vi "Parse Diff Report to Text.vi"(0 "XML Path":path, 1 "Ignore cosmetic changes? (T)":bool=TRUE, 11 "error in":errorcluster) -> (4 "change description":string, 15 "error out":errorcluster)   [LabVIEW 2020, in "Graphical Diff.lvlib"]
uses:
  Graphical Diff.lvlib
  <vilib>/xml/NI_XML.lvlib
  <resource>/objmgr/DOMUserDefRef.rc
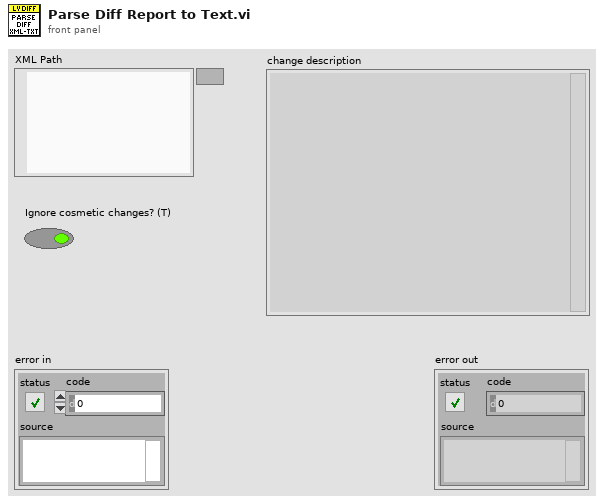
[diagram p1: front panel]
types:
  T1 = cluster{"Value":string, "Value":string, "Value":string, "Value":string}
  T2 = cluster{"Value":string, "Value":string, "Value":string, "Value":string}[]
  T3 = cluster{string, cluster{"Value":string, "Value":string, "Value":string, "Value":string}[]}
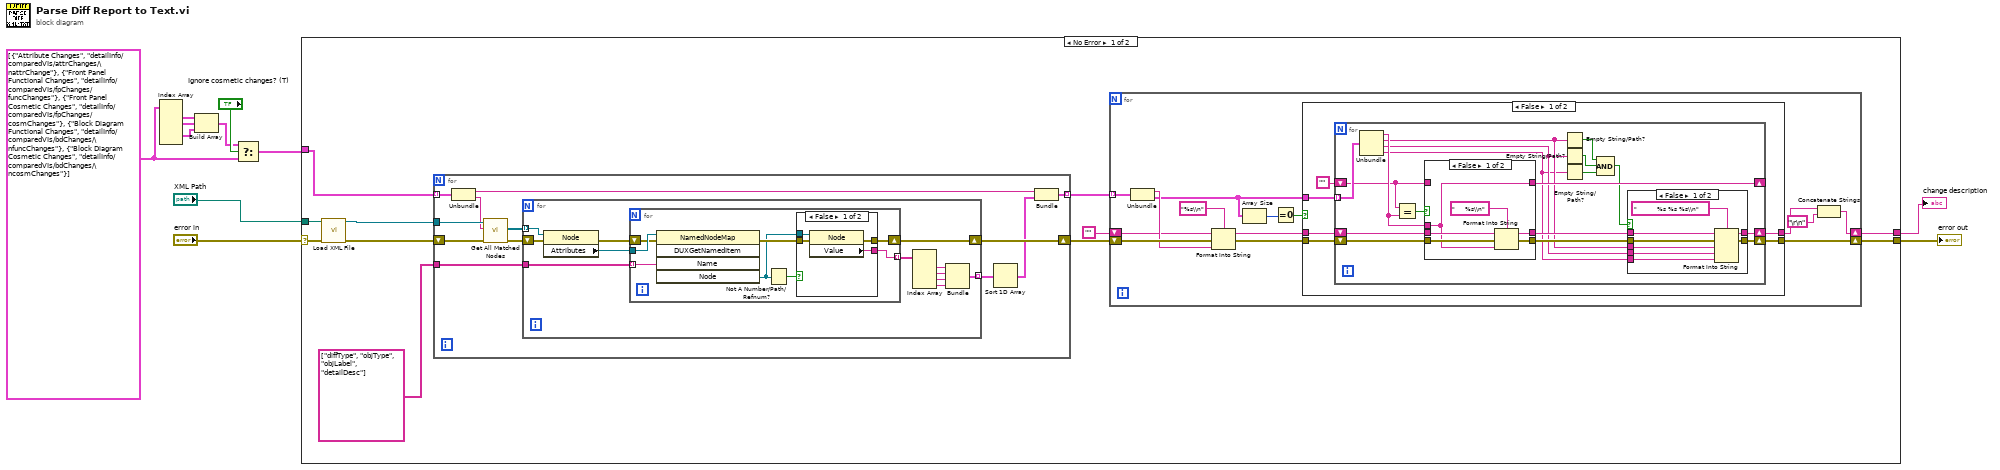
[diagram p0: block diagram]
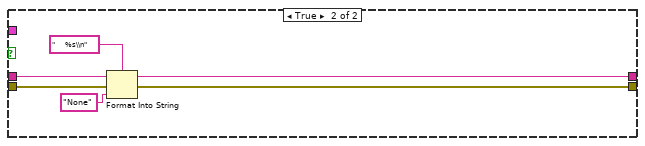
[diagram p4: hidden frame]
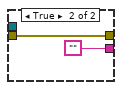
[diagram p5: hidden frame]
diagram:
  w4 = cluster{string, string}[] [{"Attribute Changes", "detailInfo/comparedVIs/attrChanges/\nattrChange"}, {"Front Panel Functional Changes", "detailInfo/comparedVIs/fpChanges/funcChanges"}, {"Front Panel Cosmetic Changes", "detailInfo/comparedVIs/fpChanges/cosmChanges"}, {"Block Diagram Functional Changes", "detailInfo/comparedVIs/bdChanges/\nfuncChanges"}, {"Block Diagram Cosmetic Changes", "detailInfo/comparedVIs/bdChanges/\ncosmChanges"}]
  n1 = Index Array(array=w4) -> (element #1=w7:cluster{string, string}, element #2=w1:cluster{string, string}, element #4=w2:cluster{string, string})  [unwired: 5 in, 2 out]
  n2 = Build Array(w7, w1, w2) -> (w5:cluster{string, string}[])
  n3 = Select(t=w5, s="Ignore cosmetic changes? (T)", f=w4) -> (s? t:f=w3:cluster{string, string}[])
  n4 = case shown="No Error" "error in" {
    selector: "error in" -> [w22 w124]
    tunnel: "XML Path" -> [w21 _]
    tunnel: [w19 w124] -> w9
    tunnel: [w18 _] -> w8
    tunnel: w3 -> [w12 _]
    frame No Error {
      n5 = call <vilib>:"Load XML File.vi"("path to XML document"=w21, "error in (no error)"=w22) -> ("DOM document out"=w17:refnum<k20>, "error out"=w16:errorcluster)  [unwired: 11 in, 1 out]
      n6 = for {
        tunnel: w17 -> [w97]
        shift-right: [w94] -> w13
        shift-left: w16 -> [w96]
        tunnel: w12 -> [w91] mode=indexing
        tunnel: string[] ["diffType", "objType", "objLabel", "detailDesc"] -> [w93]
        tunnel: [w86] -> w15 mode=indexing
        n7 = Unbundle(w91) -> (w87:string, w90:string)
        n8 = call <vilib>:"Get All Matched Nodes.vi"("error in (no error)"=w96, "XPath expression"=w90, "node in"=w97) -> ("error out"=w95:errorcluster, "node result array"=w89:refnum<k20>[])  [unwired: 6 in, 1 out]
        n9 = for {
          shift-right: [w106] -> w94
          shift-left: w95 -> [w107]
          tunnel: w93 -> [w105]
          tunnel: [w99] -> w92 mode=indexing
          tunnel: w89 -> [w98] mode=indexing
          n10 = property class="Node"(reference=w98, error in=w107) -> (error out=w109:errorcluster, "Attributes"=w108:refnum<k20>)  [unwired: 1 out]
          n11 = for {
            tunnel: w108 -> [w117]
            shift-right: [w113] -> w106
            shift-left: w109 -> [w116]
            tunnel: w105 -> [w115] mode=indexing
            tunnel: [w112] -> w104 mode=indexing
            n12 = invoke class="NamedNodeMap" method="DUXGetNamedItem"(reference=w117, error in=w116, "Name"=w115) -> (error out=w114:errorcluster, "Node"=w110:refnum<k20>)  [unwired: 2 in, 3 out]
            n13 = Not A Number/Path/Refnum?(number/path/refnum=w110) -> (NaN/Path/Refnum?=w111:bool)
            n14 = case shown="False" w111 {
              tunnel: w114 -> [w121 w123]
              tunnel: [w120 w123] -> w113
              tunnel: [w119 ""] -> w112
              tunnel: w110 -> [w118 _]
              frame False {
                n15 = property class="Node"(reference=w118, error in=w121) -> (error out=w120:errorcluster, "Value"=w119:string)  [unwired: 1 out]
              }
              frame True {
              }
            }
          }
          n16 = Index Array(array=w104) -> (element #1=w100:string, element #2=w103:string, element #3=w101:string, element #4=w102:string)  [unwired: 4 in]
          n17 = Bundle("Value"=w100, "Value"=w103, "Value"=w101, "Value"=w102) -> (w99:T1)  [unwired: 1 in]
        }
        n18 = Sort 1D Array(array=w92) -> (sorted array=w88:T2)
        n19 = Bundle(w87, w88) -> (w86:T3)  [unwired: 1 in]
      }
      n20 = for {
        tunnel: w15 -> [w36] mode=indexing
        shift-right: [w27] -> w19
        shift-left: w13 -> [w35]
        shift-right: [w24] -> w18
        shift-left: "" -> [w28]
        n21 = Unbundle(w36) -> (w34:string, w26:T2)
        n22 = Format Into String(format string="%s\\n", initial string=w28, error in=w35, w34) -> (resulting string=w29:string, error out=w30:errorcluster)
        n23 = Array Size(array=w26) -> (size(s)=w32:i32)
        n24 = Equal To 0?(x=w32) -> (x = 0?=w31:bool)
        n25 = case shown="False" w31 {
          tunnel: w30 -> [w42 w83]
          tunnel: w29 -> [w41 w82]
          tunnel: [w38 w81] -> w27
          tunnel: [w37 w80] -> w25
          tunnel: w26 -> [w40 _]
          frame False {
            n26 = for {
              shift-right: [w52] -> w38
              shift-left: w42 -> [w58]
              shift-right: [w51] -> w37
              shift-left: w41 -> [w57]
              tunnel: w40 -> [w60] mode=indexing
              shift-right: [w56] -> _
              shift-left: "" -> [w54]
              n27 = Unbundle(w60) -> ("Value"=w55:string, "Value"=w49:string, "Value"=w48:string, "Value"=w47:string)
              n28 = Equal?(x=w54, y=w55) -> (x = y?=w59:bool)
              n29 = case shown="False" w59 {
                tunnel: w58 -> [w75 w79]
                tunnel: w55 -> [w71 _]
                tunnel: w57 -> [w76 w78]
                tunnel: [w73 w79] -> w53
                tunnel: [w72 w78] -> w50
                tunnel: w54 -> [_ w77]
                tunnel: [w71 w77] -> w56
                frame False {
                  n30 = Format Into String(format string="     %s\\n", initial string=w76, error in=w75, w71) -> (resulting string=w72:string, error out=w73:errorcluster)
                }
                frame True {
                }
              }
              n31 = Empty String/Path?(string/path=w49) -> (empty?=w44:bool)
              n32 = Empty String/Path?(string/path=w48) -> (empty?=w45:bool)
              n33 = Empty String/Path?(string/path=w47) -> (empty?=w46:bool)
              n34 = Compound Arithmetic op=AND(w44, w45, w46) -> (w43:bool)
              n35 = case shown="False" w43 {
                tunnel: w53 -> [w68 w69]
                tunnel: [w67 w69] -> w52
                tunnel: [w65 w70] -> w51
                tunnel: w50 -> [w64 w70]
                tunnel: w49 -> [w63 _]
                tunnel: w48 -> [w62 _]
                tunnel: w47 -> [w61 _]
                frame False {
                  n36 = Format Into String(format string="          %s %s %s\\n", initial string=w64, error in=w68, w63, w62, w61) -> (resulting string=w65:string, error out=w67:errorcluster)
                }
                frame True {
                }
              }
            }
          }
          frame True {
            n37 = Format Into String(format string="     %s\\n", initial string=w82, error in=w83, "None" ("input 1")) -> (resulting string=w80:string, error out=w81:errorcluster)
          }
        }
        n38 = Concatenate Strings(w25, "\r\n") -> (w24:string)
      }
    }
    frame Error {
    }
  }
  "error out" <- w9
  "change description" <- w8
